vi "Read Disk Info.vi"(8 "error in (no error)":errorcluster, 11 "Linux System SAL in":refnum<class "Linux System SAL.lvclass">) -> (0 "error out":errorcluster, 3 "Linux System SAL out":refnum<class "Linux System SAL.lvclass">)   [LabVIEW 2020, in "Volatus.lvlib" / "Linux System SAL.lvclass"]
uses:
  Linux System SAL.lvclass
  Linux System SAL.lvclass/Linux System SAL.ctl
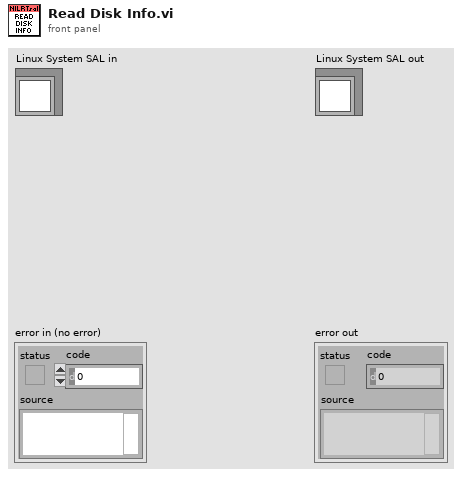
[diagram p1: front panel]
types:
  T1 = typedef "Volatus.lvlib/Linux System SAL.lvclass/Disk Info.ctl" = cluster{"Filesystem":string, "Capacity":dbl, "Used":dbl, "Available":dbl}
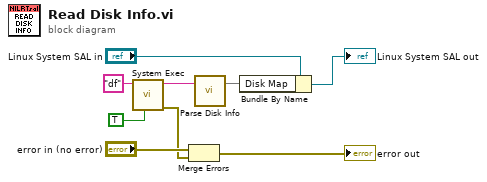
[diagram p0: block diagram]
diagram:
  n1 = call <vilib>:"System Exec.vi"("run minimized? (F)"=TRUE, "command line"="df") -> ("error out"=w1:errorcluster, "standard output"=w5:string)  [unwired: 6 in, 2 out]
  n2 = Merge Errors("error in (no error)", w1) -> (→"error out":errorcluster)
  n3 = call "Parse Disk Info.vi"("Result"=w5) -> ("Disk Map"=w3:map{string, T1})  [unwired: 6 in]
  n4 = Bundle By Name(cluster="Linux System SAL in", "Disk Map"=w3) -> (→"Linux System SAL out":refnum<class "Linux System SAL.lvclass">)
